vi "Bitstream to Bytes.vi"(8 "error in (no error)":errorcluster, 11 "bitstream":u8[](array[numeric])) -> (0 "error out":errorcluster, 3 "byte array":u8[](array[numeric]))   [LabVIEW 2013, in "GOLPI library.lvlib"]
doc: "Decodes 7-bit ascii bitstream to byte stream. Used only for decoding binary transfer via console. Coding is provided by golpi_data2bits.m in octave package golpi. Error in is passed through to error out without changes."
uses:
  GOLPI library.lvlib
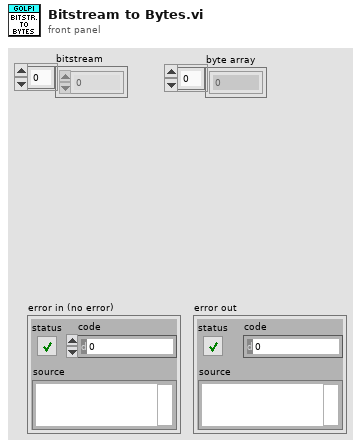
[diagram p1: front panel]
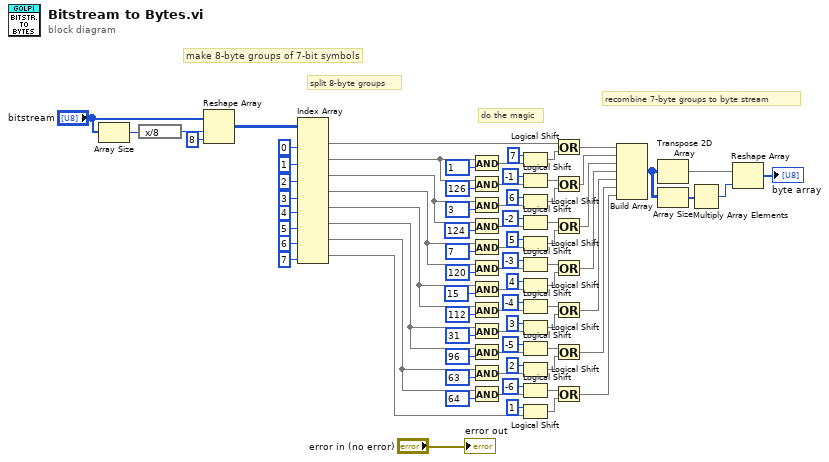
[diagram p0: block diagram]
diagram:
  # "recombine 7-byte groups to byte stream"
  # "do the magic"
  # "split 8-byte groups"
  # "make 8-byte groups of 7-bit symbols"
  n1 = Array Size(array="bitstream") -> (size(s)=w1:i32)
  n2 = expression code="x/8"(w1) -> (w2:i32)
  n3 = Reshape Array("bitstream", w2, 8 ("dimension size")) -> (w82:u8[][])
  n4 = Index Array(array=w82, index (col) #1=0 ("disabled index (col)"), index (col) #2=1 ("index (col)"), index (col) #3=2 ("index (col)"), index (col) #4=3 ("index (col)"), index (col) #5=4 ("index (col)"), index (col) #6=5 ("index (col)"), index (col) #7=6 ("index (col)"), index (col) #8=7 ("index (col)")) -> (element #1=w71:u8[], element #2=w67:u8[], element #3=w51:u8[], element #4=w42:u8[], element #5=w33:u8[], element #6=w24:u8[], element #7=w17:u8[], element #8=w5:u8[])  [unwired: 8 in]
  n5 = And(x=w67, y=u8 1 ("dimension size")) -> (x .and. y?=w68:u8[])
  n6 = And(x=w67, y=u8 126 ("dimension size")) -> (x .and. y?=w66:u8[])
  n7 = And(x=w51, y=u8 3 ("dimension size")) -> (x .and. y?=w62:u8[])
  n8 = And(x=w51, y=u8 124 ("dimension size")) -> (x .and. y?=w54:u8[])
  n9 = And(x=w42, y=u8 7 ("dimension size")) -> (x .and. y?=w57:u8[])
  n10 = And(x=w42, y=u8 120 ("dimension size")) -> (x .and. y?=w48:u8[])
  n11 = And(x=w33, y=u8 15 ("dimension size")) -> (x .and. y?=w45:u8[])
  n12 = And(x=w33, y=u8 112 ("dimension size")) -> (x .and. y?=w36:u8[])
  n13 = And(x=w24, y=u8 31 ("dimension size")) -> (x .and. y?=w39:u8[])
  n14 = And(x=w24, y=u8 96 ("dimension size")) -> (x .and. y?=w30:u8[])
  n15 = And(x=w17, y=u8 63 ("dimension size")) -> (x .and. y?=w27:u8[])
  n16 = And(x=w17, y=u8 64 ("dimension size")) -> (x .and. y?=w20:u8[])
  n17 = Logical Shift(y=i16 7, x=w68) -> (x << y=w70:u8[])
  n18 = Logical Shift(y=i16 -1, x=w66) -> (x << y=w61:u8[])
  n19 = Logical Shift(y=i16 6, x=w62) -> (x << y=w60:u8[])
  n20 = Logical Shift(y=i16 -2, x=w54) -> (x << y=w58:u8[])
  n21 = Logical Shift(y=i16 5, x=w57) -> (x << y=w59:u8[])
  n22 = Logical Shift(y=i16 -3, x=w48) -> (x << y=w44:u8[])
  n23 = Logical Shift(y=i16 4, x=w45) -> (x << y=w43:u8[])
  n24 = Logical Shift(y=i16 -4, x=w36) -> (x << y=w40:u8[])
  n25 = Logical Shift(y=i16 3, x=w39) -> (x << y=w41:u8[])
  n26 = Logical Shift(y=i16 -5, x=w30) -> (x << y=w26:u8[])
  n27 = Logical Shift(y=i16 2, x=w27) -> (x << y=w25:u8[])
  n28 = Logical Shift(y=i16 -6, x=w20) -> (x << y=w22:u8[])
  n29 = Logical Shift(y=i16 1, x=w5) -> (x << y=w23:u8[])
  n30 = Or(x=w71, y=w70) -> (x .or. y?=w16:u8[])
  n31 = Or(x=w61, y=w60) -> (x .or. y?=w15:u8[])
  n32 = Or(x=w58, y=w59) -> (x .or. y?=w14:u8[])
  n33 = Or(x=w44, y=w43) -> (x .or. y?=w13:u8[])
  n34 = Or(x=w40, y=w41) -> (x .or. y?=w12:u8[])
  n35 = Or(x=w26, y=w25) -> (x .or. y?=w11:u8[])
  n36 = Or(x=w22, y=w23) -> (x .or. y?=w10:u8[])
  n37 = Build Array(w16, w15, w14, w13, w12, w11, w10) -> (w8:u8[][])
  n38 = Transpose 2D Array(2D array=w8) -> (transposed array=w9:u8[][])
  n39 = Array Size(array=w8) -> (size(s)=w7:i32[])
  n40 = Multiply Array Elements(1:w7) -> (0:w6:i32)
  n41 = Reshape Array(w9, w6) -> (→"byte array":u8[])
  "error out" <- "error in (no error)"
